vi "Test-DotNet-directLogin.vi"() -> ()   [LabVIEW 2013, in "HardwareCharacterization.lvlib" / "HC-SM1000.lvclass"]
uses:
  HC-SM1000.lvclass
  DOTNET-settings.ctl
  Device-identification.ctl
  Fixed-data-type.ctl
panel:
  out "Job count":i32
  out "Job name list":string
  out "Fixed data":string
  in  "File name wo extension":string="AdminConfig"
  in  "Fixed data type":T1=10 items=["Controller Configuration"=5, "Laser Configuration"=6, "Lens Configuration"=2, "Correction Table"=13, "User Configuration"=15, "Performance Adjustments"=16, "Admin Configuration"=10]
  in  "Device index":i32
  in  "DOTNET settings":T2={"Target IP"="128.178.146.163", "Target broadcast port"=11000, "Target communication port"=12200, "clientID"=-1, "Broadcast IP"="224.168.100.2", "Servercount"=-1, "Device IDs"=[{"Name"="EC1000", "IP"="128.178.146.163", "Mac address"="mac"}]}
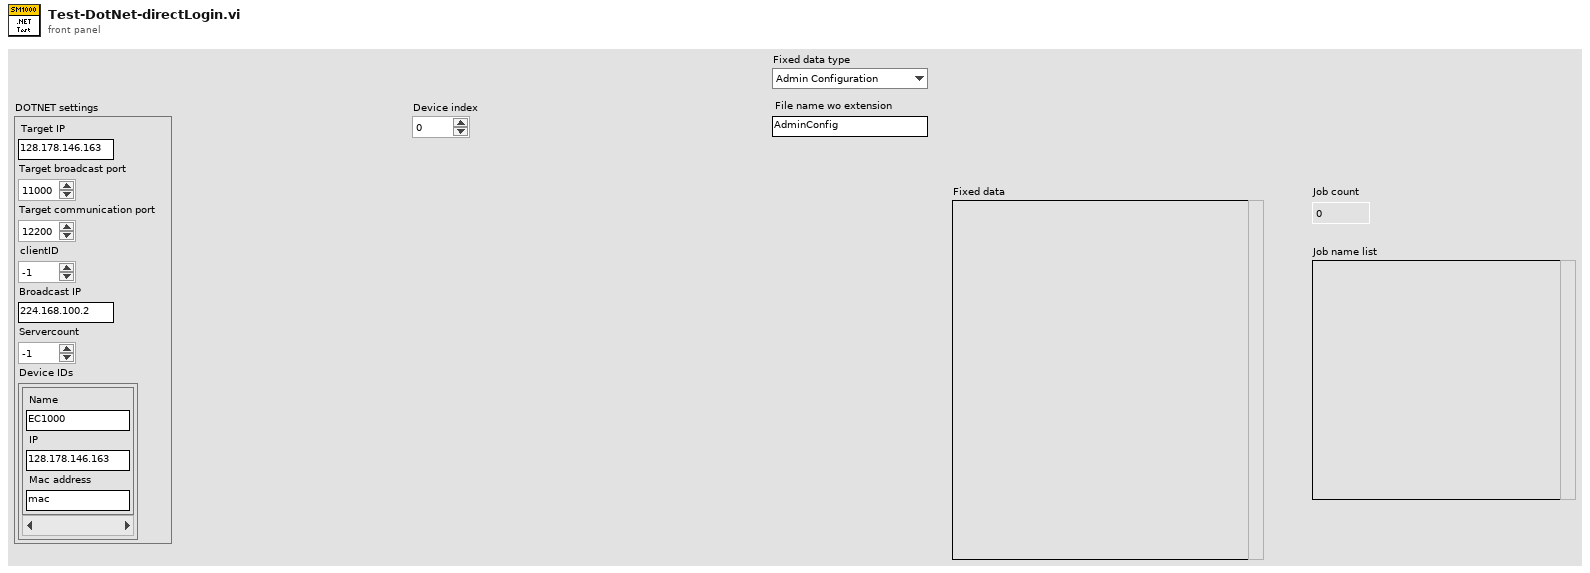
[diagram p1: front panel]
types:
  T1 = typedef "HardwareCharacterization.lvlib/HC-SM1000.lvclass/Fixed-data-type.ctl" = i32
  T2 = typedef "HardwareCharacterization.lvlib/HC-SM1000.lvclass/DOTNET-settings.ctl" = cluster{"Target IP":string, "Target broadcast port":i32, "Target communication port":i32, "clientID":i32, "Broadcast IP":string, "Servercount":i32, "Device IDs":T3[]}
  T3 = typedef "HardwareCharacterization.lvlib/HC-SM1000.lvclass/Device-identification.ctl" = cluster{"Name":string, "IP":string, "Mac address":string}
  T4 = typedef "HardwareCharacterization.lvlib/HC-SM1000.lvclass/Object-reference.ctl" = refnum<data-value>
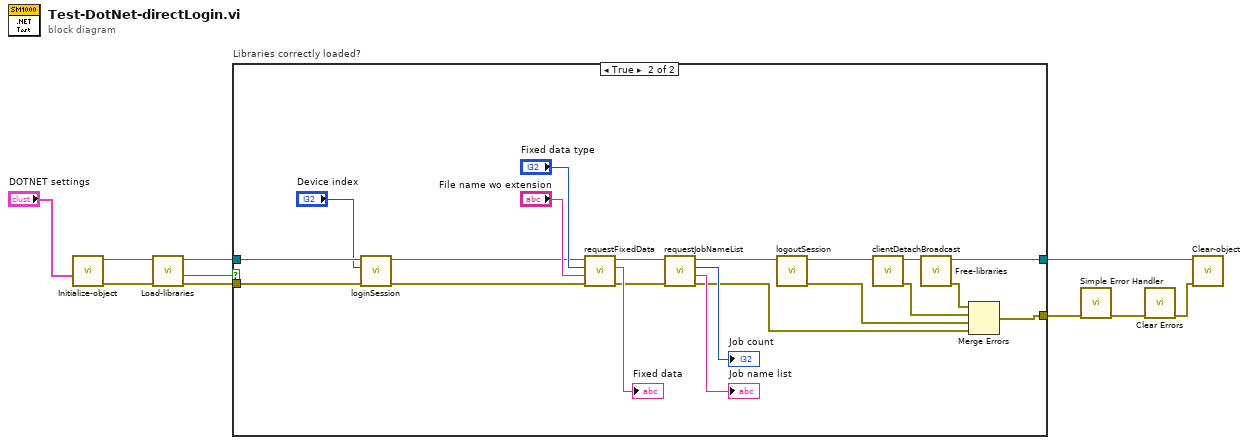
[diagram p0: block diagram]
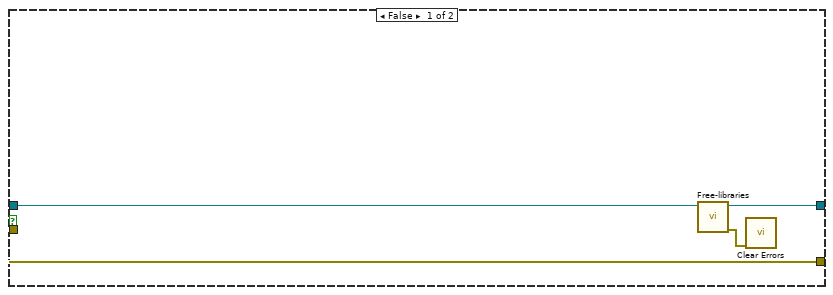
[diagram p2: hidden frame]
diagram:
  n1 = call "Initialize-object.vi"("DOTNET settings"="DOTNET settings") -> ("error out"=w8:errorcluster, "SM1000-control out"=w9:T4)  [unwired: 9 in]
  n2 = call "Load-libraries.vi"("error in (no error)"=w8, "SM1000-control in"=w9) -> ("error out"=w5:errorcluster, "Loaded?"=w7:bool, "SM1000-control out"=w6:T4)  [unwired: 7 in]
  n3 = case "Libraries correctly loaded?" shown="True" w7 {
    tunnel: w6 -> [w13 w28]
    tunnel: w5 -> [w14 w27]
    tunnel: [w14 w34] -> w3
    tunnel: [w12 w33] -> w1
    frame False {
      n4 = call "Free-libraries.vi"("SM1000-control in"=w13) -> ("error out"=w11:errorcluster, "SM1000-control out"=w12:T4)  [unwired: 8 in, 1 out]
      n5 = call <vilib>:"Clear Errors.vi"("error in (no error)"=w11) -> ()  [unwired: 6 in, 1 out]
    }
    frame True {
      n6 = call "loginSession.vi"("error in (no error)"=w27, "Device index"="Device index", "SM1000-control in"=w28) -> ("error out"=w23:errorcluster, "SM1000-control out"=w24:T4)  [unwired: 7 in]
      n7 = call "requestFixedData.vi"("error in (no error)"=w23, "File name wo extension"="File name wo extension", "Fixed data type"="Fixed data type", "SM1000-control in"=w24) -> ("error out"=w20:errorcluster, "File contents"=→"Fixed data":string, "SM1000-control out"=w21:T4)  [unwired: 5 in]
      n8 = call "requestJobNameList.vi"("error in (no error)"=w20, "SM1000-control in"=w21) -> ("error out"=w15:errorcluster, "Job name list"=→"Job name list":string, "Job count"=→"Job count":i32, "SM1000-control out"=w19:T4)  [unwired: 6 in]
      n9 = call "logoutSession.vi"("SM1000-control in"=w19) -> ("error out"=w30:errorcluster, "SM1000-control out"=w29:T4)  [unwired: 9 in]
      n10 = call "clientDetachBroadcast.vi"("SM1000-control in"=w29) -> ("error out"=w31:errorcluster, "SM1000-control out"=w32:T4)  [unwired: 9 in]
      n11 = call "Free-libraries.vi"("SM1000-control in"=w32) -> ("error out"=w35:errorcluster, "SM1000-control out"=w33:T4)  [unwired: 8 in, 1 out]
      n12 = Merge Errors(w35, w31, w30, w15) -> (w34:errorcluster)
    }
  }
  n13 = call <vilib>:"Simple Error Handler.vi"("error in (no error)"=w3) -> ("error out"=w4:errorcluster)  [unwired: 4 in, 4 out]
  n14 = call <vilib>:"Clear Errors.vi"("error in (no error)"=w4) -> ("error out"=w2:errorcluster)  [unwired: 6 in]
  n15 = call "Clear-object.vi"("error in (no error)"=w2, "SM1000-control"=w1) -> ()  [unwired: 8 in, 2 out]
